vi "Filename Sanitizer.vi"(10 "Replace String (_)":string="_", 11 "String in":string) -> (3 "String out":string)   [LabVIEW 2022 SP3, in "hse-misc.lvlib"]
doc: "Removes all characters that are not supported in filenames (/ \\ : * ? \" < > | ) and replaces it with \"Replace String\" (default is \"_\").\n\n____\nHAMPEL SOFTWARE ENGINEERING v3.8.0 (2023-12-18 14:41)"
uses:
  hse-misc.lvlib
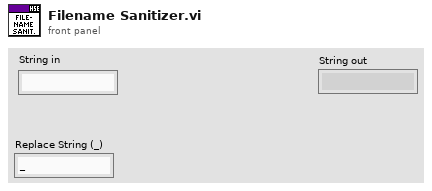
[diagram p1: front panel]
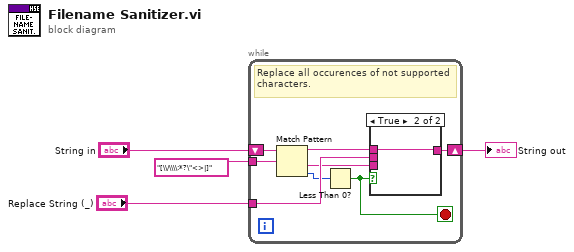
[diagram p0: block diagram]
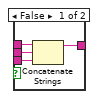
[diagram p2: hidden frame]
diagram:
  n1 = while {
    tunnel: "[\\/\\\\:*?\"<>|]" -> [w11]
    shift-right: [w7] -> w1
    shift-left: "String in" -> [w12]
    tunnel: "Replace String (_)" -> [w9]
    stop <- w5 stop-if-true
    # "Replace all occurences of not supported characters."
    n2 = Match Pattern(string=w12, regular expression=w11) -> (before substring=w10:string, after substring=w8:string, offset past match=w6:i32)  [unwired: 1 in, 1 out]
    n3 = Less Than 0?(x=w6) -> (x < 0?=w5:bool)
    n4 = case shown="True" w5 {
      tunnel: w10 -> [w16 w17]
      tunnel: w9 -> [w15 _]
      tunnel: w8 -> [w14 _]
      tunnel: [w13 w17] -> w7
      frame False {
        n5 = Concatenate Strings(w16, w15, w14) -> (w13:string)
      }
      frame True {
      }
    }
  }
  "String out" <- w1
